vi "Distance between 2 frame.vi"(10 "Goal Frame (World)":cluster{"X":sgl, "Y":sgl, "Theta":dbl}, 11 "Robot Frame (World)":cluster{"X":sgl, "Y":sgl, "Theta":dbl}) -> (3 "sqrt(x)":sgl)   [LabVIEW 2016]
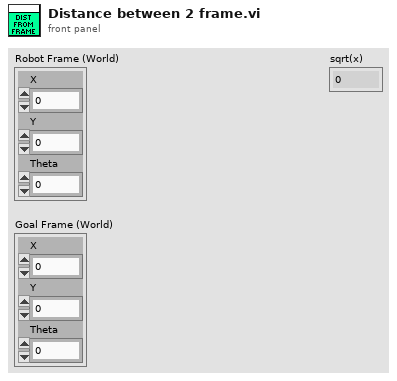
[diagram p1: front panel]
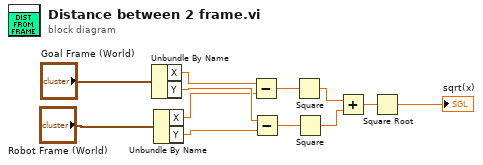
[diagram p0: block diagram]
diagram:
  n1 = Unbundle By Name("Goal Frame (World)") -> ("X"=w4:sgl, "Y"=w6:sgl)
  n2 = Unbundle By Name("Robot Frame (World)") -> ("X"=w5:sgl, "Y"=w7:sgl)
  n3 = Subtract(x=w4, y=w5) -> (x-y=w8:sgl)
  n4 = Subtract(x=w6, y=w7) -> (x-y=w9:sgl)
  n5 = Square(x=w8) -> (x^2=w10:sgl)
  n6 = Square(x=w9) -> (x^2=w11:sgl)
  n7 = Add(x=w10, y=w11) -> (x+y=w12:sgl)
  n8 = Square Root(x=w12) -> (sqrt(x)=→"sqrt(x)":sgl)
